vi "AlliGator Is Search ROI Modified.vi"(8 "Error In":errorcluster, 11 "Display Image Control Refnum":T1) -> (0 "Error Out":errorcluster, 3 "Search ROI Changed":bool)   [LabVIEW 2021, in "AlliGator Source Image.lvlib"]
doc: "If the \"Use Search ROI\" option is checked and the user modified the ROI, uncheck this option."
uses:
  AlliGator Source Image.lvlib
  Image/Image Control Refnum.ctl
  Globals, Variables, Constants/AlliGator Variables List.ctl
  Variant/Variant to Data/Variant to Boolean.vi
  Globals, Variables, Constants/AlliGator Globals, Variables & Constants.lvlib
  Variant/Variant to Data/Variant to Data.lvlib
  Image/Image.lvlib
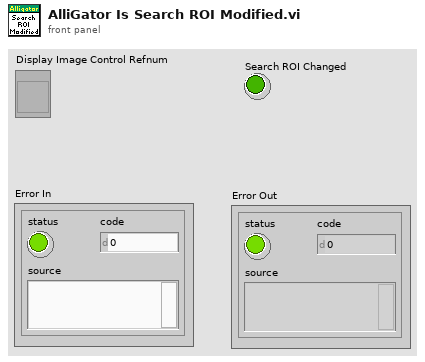
[diagram p1: front panel]
types:
  T1 = typedef "Image.lvlib/Image Control Refnum.ctl" = refnum<vi>
  T2 = typedef "AlliGator Globals, Variables & Constants.lvlib/AlliGator Variables List.ctl" = enum16{"---- GUI ----", "GUI:Initialization Status", "GUI:State Indicators Refnum", "GUI:Original AlliGator Menu Items", "GUI:Current Action Loop State", "GUI:Script in progress", "GUI:Playback", "GUI:Loop Playback", "GUI:Search ROI Used", "GUI:Search ROI", "Decay Graph Max Legend Size", "Intensity Graph Max Legend Size", "Decay Statistics Graph Max Legend Size", "Phasor Graph Max Legend Size", "Phasor Ratio Graph Max Legend Size", "Lifetime Graph Max Legend Size", "---- Files ----", "Files:Export Dataset Frames as Individual Files", "Files:Show Batch Export Help Balloons", "Files:Frames in Dataset", "Files:ptu File Frame Start Indices", "Files:Current Frame in Dataset", "Files:Current Frame Timestamp", "Files:Dataset Loaded", "Files:Dataset Metadata", "Files:Dataset Channel", "Files:Dataset Data Description", "Files:Background Dataset Metadata", "Files:Background Dataset Channel", "Files:Background Dataset Data Description", "Files:Background File Subtraction", "Files:Background File Path", "Files:Background File Pile-up Correction", "Files:Background File Pixel Well Capacity", "Files:Background File Scaling Factor", "Files:Current Dataset Load Settings", "Files:Dataset Path", "Files:ICCD-specific Information", "Files:Macrotime Gate Separation", "------ Python Plugins ------", "Python Plugins:Information", "Python Plugins:Python Session", "Python Plugins:Valid Python Session?", "---- Source Image ----", "Source Image:ROIs", "Source Image:Current ROI", "Source Image:ROI Event Refnum", "X_Source Image Display Range", "X_Source Image Palette Information", "X_Type of Displayed Image", "X_Time Gate Slider", "Source Image:Palette List", "Source Image:Scale", "Source Image:ROI Overlay Color", "Source Image:Overlay to Erase", "Source Image:Is Displayed Image Accumulated", "Source Image:White Light Image Modified", "Source Image:Mask Image Modified", "---- Image Profile Window ----", "Image Profile:Window Event Refnum", "Image Profile:IntensityType", "Image Profile:Intensity Average Type", "Image Profile:Intensity-weighted SDV", "Image Profile:Box Profile Type", "Image Profile:Window Open", "Image Profile:Plotted Fit Parameter", "------ Phasor Graph -------", "Phasor Graph:Show Line", "---- Phasor Plot ---", "Phasor Plot:Parameters Changed", "Phasor Plot:FLI Dataset Modified since last Calculation", "Phasor Harmonics Data", "Selected Phasor Harmonics", "Phasor Harmonic Manager Event Refnum", "Phasor Plot:ROIs", "Phasor Plot:Current ROI", "Phasor Plot:ROI Event Refnum", "Phasor Plot:Image Reference Points", "Phasor Plot:Computed", "Phasor Plot:Palette Information", "Phasor Plot:Palette List", "Phasor Plot:Phasor Ratio Palette Information", "Phasor Plot:Phasor Ratio Palette List", "Phasor Plot:Image Scale", "Phasor Plot:Image Overlay to Erase", "Phasor Plot:Image Elements to Update", "Phasor Plot:Current Calculation Parameters", "Phasor Plot:Current Calibration Options", "Phasor Plot:Reset Cumulated Phasor Plot", "Phasor Plot:Reference 1", "Phasor Plot:Lifetime Reference 1", "Phasor Plot:Reference 1 Frequency", "Phasor Plot:Reference 2", "Phasor Plot:Lifetime Reference 2", "Phasor Plot:Reference 2 Frequency", "---- Decay Analysis ----", "Number of Selected Decays to Fit", "LS Fit Results", "LAR Fit Results", "BS Fit Results", "Last Decay Max - Min", "Best Fit Parameters", "Best Fit Parameter Names", "Actual Size X", "Actual Size Y", "Binning X", "Binning Y", "Actual # Gates", "Dataset Number", "Gates to...", "Gates Skipped", "Gates to keep", "Gate Step", "Gate Separation", "Reversed Gates", "Pile-up Correction", "Pixel Well Capacity", "Background Subtracted", "Background Subtraction Method", "Background Definition Range", "Background File (deprecated)", "Number of Dataset Accumulated", "Array of Accumulated Dataset Paths", "Do Averaged Datasets", "Destination File Path", "Process Plot Target", "Use 1/D as Phasor Frequency", "---- Decay Fit Parameter Map -----", "Decay Fit Parameter Map:Palette Information", "Decay Fit Parameter Map:Palette List", "---- Parameter Map ----", "Parameter Map:Palette Information", "Parameter Map:Palette List", "------- Local Decay Window ---------", "Local Decay Graph Window:Event Refnum", "Local Decay Graph Window:Use normalized IRF for convolution", "----- Miscellaneous ----", "Misc:Skippable Dialog Windows Status"}
  T3 = cluster{"Global Rectangle":i32[], "Contours":cluster{"Contour Type":u32, "ROI Type":u32, "Points":i32[]}[]}
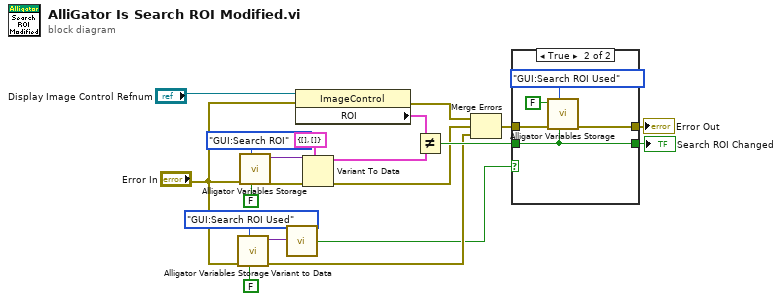
[diagram p0: block diagram]
diagram:
  n1 = call "Alligator Variables Storage.vi"("Get(F)/Set"=FALSE, "AlliGator Variable"=AlliGator_Variables_List."GUI:Search ROI Used" ("Alligator Variable"), "Error In"="Error In") -> ("Error Out"=w3:errorcluster, "Data out"=w4:variant)  [unwired: 6 in, 1 out]
  n2 = call "Alligator Variables Storage.vi"("Get(F)/Set"=FALSE, "AlliGator Variable"=AlliGator_Variables_List."GUI:Search ROI" ("Alligator Variable"), "Error In"="Error In") -> ("Error Out"=w17:errorcluster, "Data out"=w18:variant)  [unwired: 6 in, 1 out]
  n3 = call-poly "Variant to Data.vi"("Variant"=w4) -> ("Value"=w2:bool)  [unwired: 8 in]
  n4 = property class="ImageControl"(reference="Display Image Control Refnum", error in="Error In") -> (error out=w8:errorcluster, "ROI"=w16:T3)  [unwired: 1 out]
  n5 = Variant To Data(error in=w17, type=T3 {"Global Rectangle"=[], "Contours"=[]} ("ROI"), Variant=w18) -> (data=w15:T3, error out=w10:errorcluster)
  n6 = Not Equal?(x=w16, y=w15) -> (x != y?=w13:bool)
  n7 = Merge Errors(w8, w10, w3) -> (w9:errorcluster)
  n8 = case shown="True" w2 {
    selector: w2 -> [w21 _]
    tunnel: w13 -> [_ w23]
    tunnel: [w22 w26] -> w11
    tunnel: w9 -> [w22 w25]
    tunnel: [w21 w23] -> w1
    frame False {
    }
    frame True {
      n9 = call "Alligator Variables Storage.vi"("Get(F)/Set"=w23, "AlliGator Variable"=AlliGator_Variables_List."GUI:Search ROI Used" ("Alligator Variable"), "Error In"=w25, "Data in"=FALSE ("x != y?")) -> ("Error Out"=w26:errorcluster)  [unwired: 5 in, 2 out]
    }
  }
  "Error Out" <- w11
  "Search ROI Changed" <- w1
